vi "Fpga-Pulse.vi"(11 "AXI_STR_TXD_tready":bool) -> (3 "Boolean":bool)   [LabVIEW 2017]
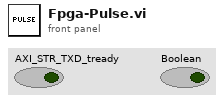
[diagram p1: front panel]
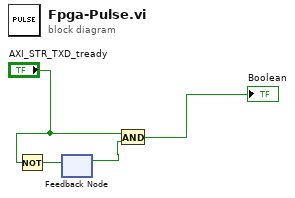
[diagram p0: block diagram]
diagram:
  n1 = Not(x="AXI_STR_TXD_tready") -> (.not. x?=w3:bool)
  n2 = feedback #1() -> (w1:bool)  [unwired: 1 in]
  n3 = feedback-in #1(w3) -> ()
  n4 = And(x="AXI_STR_TXD_tready", y=w1) -> (x .and. y?=→"Boolean":bool)
